vi "Delete Source Tags.vi"(8 "error in (no error)":errorcluster, 11 "BuildSpec in":refnum<vi>) -> (0 "error out":errorcluster, 3 "BuildSpec out":refnum<vi>)   [LabVIEW 2019, in "Project Sync Tools.lvclass"]
uses:
  Project Sync Tools.lvclass
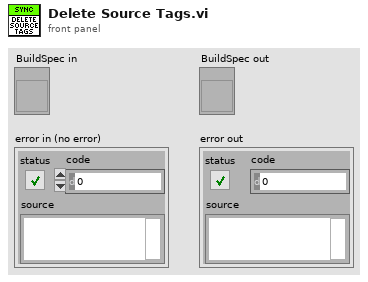
[diagram p1: front panel]
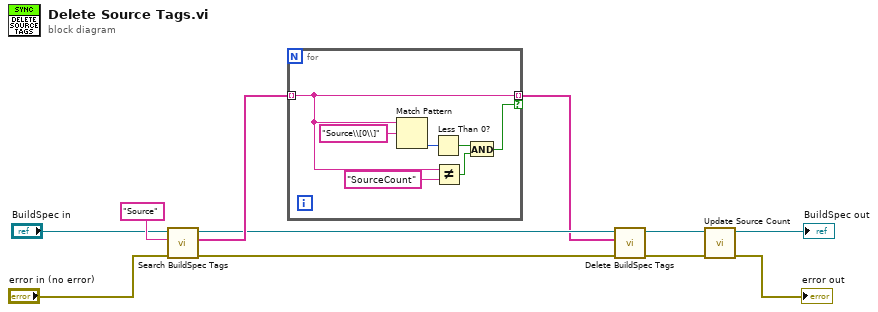
[diagram p0: block diagram]
diagram:
  n1 = call "Search BuildSpec Tags.vi"("error in (no error)"="error in (no error)", "Regular expression"="Source", "BuildSpec in"="BuildSpec in") -> ("error out"=w7:errorcluster, "Tag Names"=w8:string[], "BuildSpec out"=w6:refnum<vi>)  [unwired: 6 in]
  n2 = for {
    tunnel: w8 -> [w15] mode=indexing
    tunnel: [w15] -> w5 mode=indexing if=w12
    n3 = Match Pattern(string=w15, regular expression="Source\\[0\\]") -> (offset past match=w17:i32)  [unwired: 1 in, 3 out]
    n4 = Less Than 0?(x=w17) -> (x < 0?=w13:bool)
    n5 = Not Equal?(x=w15, y="SourceCount" ("regular expression")) -> (x != y?=w14:bool)
    n6 = And(x=w13, y=w14) -> (x .and. y?=w12:bool)
  }
  n7 = call "Delete BuildSpec Tags.vi"("error in (no error)"=w7, "Tag Names"=w5, "ProjectItem in"=w6) -> ("error out"=w4:errorcluster, "ProjectItem out"=w3:refnum<vi>)  [unwired: 6 in, 1 out]
  n8 = call "Update Source Count.vi"("error in (no error)"=w4, "BuildSpec in"=w3) -> ("error out"=→"error out":errorcluster, "BuildSpec out"=→"BuildSpec out":refnum<vi>)  [unwired: 8 in]
